vi "arduinoDetachAllServos.vi"   [LabVIEW 2012]
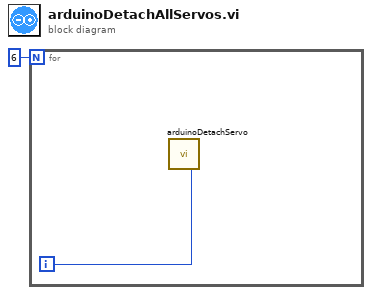
[diagram p0: block diagram]
diagram:
  n1 = for {
    N: 6 -> [_]
    i -> [w2]
    n2 = call "arduinoDetachServo.vi"("channel"=w2) -> ()
  }
